vi "HandleServers.vi"(8 "error in (no error)":errorcluster, 11 "S4ACS_GUI in":refnum<class "GuiderSetup.lvclass">) -> (0 "error out":errorcluster, 3 "S4ACS_GUI out":refnum<class "GuiderSetup.lvclass">)   [LabVIEW 2018, in "GuiderSetup.lvclass"]
uses:
  GuiderSetup.lvclass
  C:/Users/observer/Desktop/Sparc4GUI/Versao ZeroMQ/SPARC4_GUI/S4GUI/S4GUI.lvclass
  S4GUI/S4GUI.lvclass/S4GUI.ctl
  GuiderSetup.lvclass/GuiderSetup.ctl
  Instrument/Instrument.lvclass
  AG/AG.lvclass
  S4GUI/S4GUI.lvclass
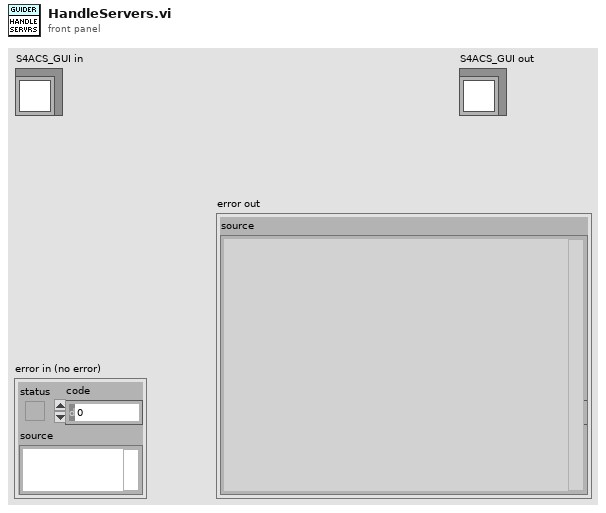
[diagram p1: front panel]
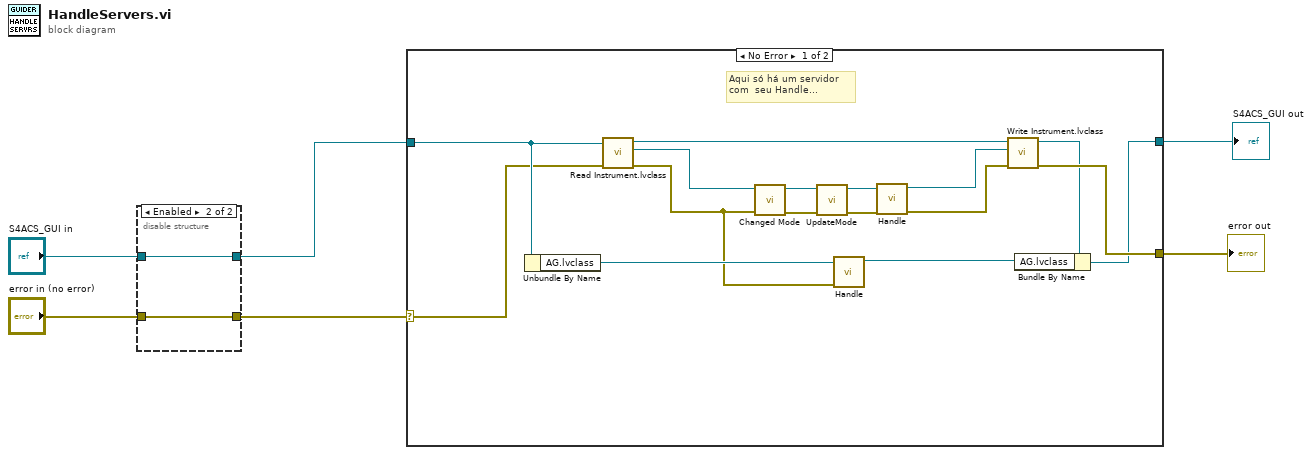
[diagram p0: block diagram]
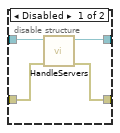
[diagram p3: hidden frame]
diagram:
  n1 = disable-structure shown="Enabled" {
    disable-tunnel: [w10 w11] -> w3
    disable-tunnel: [w9 w12] -> w4
    disable-tunnel: "error in (no error)" -> [w8 w11]
    disable-tunnel: "S4ACS_GUI in" -> [w7 w12]
    frame Disabled {
      n2 = call-parent "HandleServers.vi"("error in (no error)"=w8, "S4GUI in"=w7) -> ("error out"=w10:errorcluster, "S4GUI out"=w9:refnum<class "GuiderSetup.lvclass">)  [unwired: 8 in]
    }
    frame Enabled {
    }
  }
  n3 = case shown="No Error" w3 {
    selector: w3 -> [w23 w30]
    tunnel: [w26 w30] -> w1
    tunnel: [w19 w29] -> w2
    tunnel: w4 -> [w24 w29]
    frame No Error {
      # "Aqui só há um servidor \ncom  seu Handle..."
      n4 = Unbundle By Name(w24) -> ("AG.lvclass"=w22:refnum<class "AG.lvclass">)
      n5 = call "Read Instrument.lvclass.vi"("error in (no error)"=w23, "S4ACS_GUI in"=w24) -> ("error out"=w15:errorcluster, "Instrument.lvclass"=w18:refnum<class "Instrument.lvclass">, "S4ACS_GUI out"=w25:refnum<class "GuiderSetup.lvclass">)  [unwired: 7 in]
      n6 = call-dynamic "Changed Mode.vi"("error in (no error)"=w15, "Instrument in"=w18) -> ("error out"=w14:errorcluster, "Instrument out"=w17:refnum<class "Instrument.lvclass">)  [unwired: 8 in]
      n7 = call-dynamic "UpdateMode.vi"("error in (no error)"=w14, "Instrument in"=w17) -> ("error out"=w13:errorcluster, "Instrument out"=w16:refnum<class "Instrument.lvclass">)  [unwired: 8 in]
      n8 = call-dynamic "Handle.vi"("error in (no error)"=w15, "AG in"=w22) -> ("AG out"=w21:refnum<class "AG.lvclass">)  [unwired: 8 in, 1 out]
      n9 = call-dynamic "Handle.vi"("error in (no error)"=w13, "Instrument in"=w16) -> ("error out"=w27:errorcluster, "Instrument out"=w28:refnum<class "Instrument.lvclass">)  [unwired: 8 in]
      n10 = call "Write Instrument.lvclass.vi"("error in (no error)"=w27, "Instrument.lvclass"=w28, "S4ACS_GUI in"=w25) -> ("error out"=w26:errorcluster, "S4ACS_GUI out"=w20:refnum<class "GuiderSetup.lvclass">)  [unwired: 7 in]
      n11 = Bundle By Name(cluster=w20, "AG.lvclass"=w21) -> (w19:refnum<class "GuiderSetup.lvclass">)
    }
    frame Error {
    }
  }
  "error out" <- w1
  "S4ACS_GUI out" <- w2
